vi "Read configuration.vi"(8 "error in":errorcluster, 11 "Getting Started IO editor node in":refnum<class "io editor node.lvclass">) -> (0 "error out":errorcluster, 2 "configuration":refnum<class "NISE_CEF_serializable configuration.lvclass">, 3 "Getting Started IO editor node out":refnum<class "io editor node.lvclass">)   [LabVIEW 2014, in "io editor node.lvclass"]
uses:
  io editor node.lvclass
  <vilib>/NI/Configuration Framework/serializable configuration/NISE_CEF_serializable configuration.lvclass
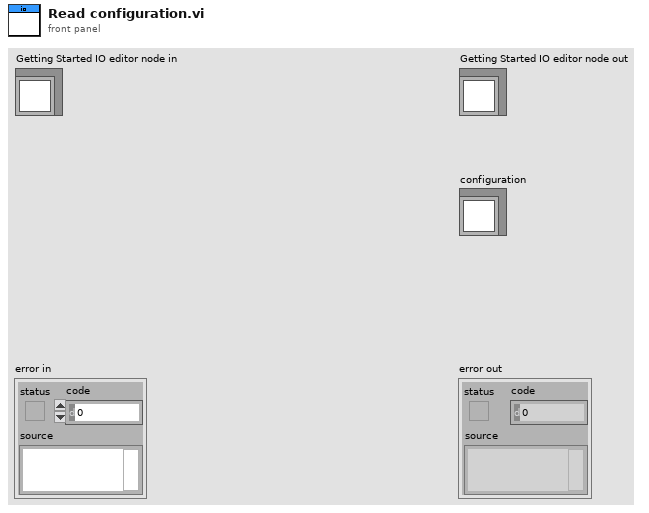
[diagram p1: front panel]
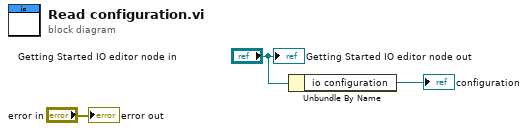
[diagram p0: block diagram]
diagram:
  n1 = Unbundle By Name("Getting Started IO editor node in") -> ("io configuration"=→"configuration":refnum<class "io configuration.lvclass">)
  "error out" <- "error in"
  "Getting Started IO editor node out" <- "Getting Started IO editor node in"
